vi "SCMP - limit FPS.vi"(7 "circural buffer?":bool, 10 "Max FPS limit in":dbl, 11 "FPS in":dbl) -> (3 "FPS out":dbl)   [LabVIEW 2014]
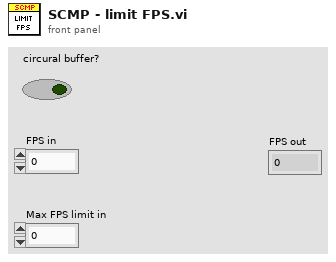
[diagram p1: front panel]
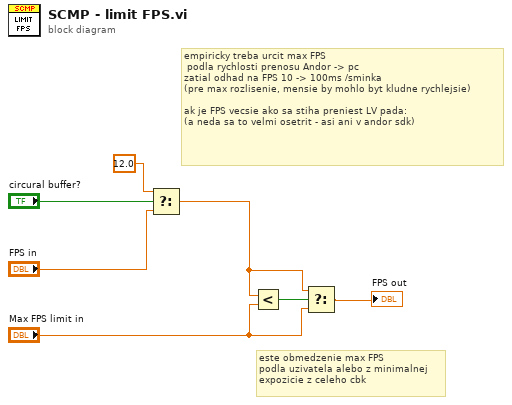
[diagram p0: block diagram]
diagram:
  # "este obmedzenie max FPS \npodla uzivatela alebo z minimalnej \nexpozicie z celeho cbk"
  # "empiricky treba urcit max FPS\n podla rychlosti prenosu Andor -> pc\nzatial odhad na FPS 10 -> 100ms /sminka\n(pre max rozlisenie, mensie by mohlo byt kludne rychlejsie)\n\nak je FPS vecsie ako sa stiha preniest LV pada:\n(a neda sa to velmi osetrit - asi ani v andor sdk)"
  n1 = Select(t=12.0, s="circural buffer?", f="FPS in") -> (s? t:f=w2:dbl)
  n2 = Less?(x=w2, y="Max FPS limit in") -> (x < y?=w5:bool)
  n3 = Select(t=w2, s=w5, f="Max FPS limit in") -> (s? t:f=→"FPS out":dbl)
